vi "Feature_flower(SubVI).vi"(4 "黄色分量（油菜花）二值图":T1) -> (0 "SF 3":dbl, 1 "IFD 2":sgl, 2 "SFD 2":sgl, 3 "SH 2":dbl, 5 "SW 2":dbl, 7 "SE 2":dbl, 8 "SA":dbl)   [LabVIEW 2015]
uses:
  <vilib>/vision/Image Controls.llb/IMAQ Image.ctl
  <vilib>/vision/NI_Vision_Development_Module.lvlib
  2-top_features_oilseed/fractaldim.dll
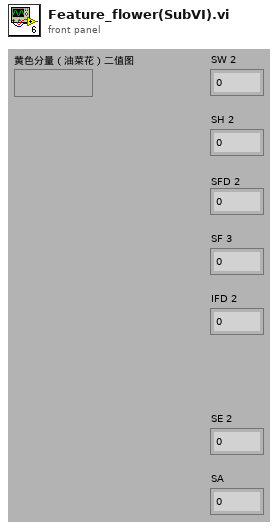
[diagram p1: front panel]
types:
  T1 = typedef "IMAQ Image.ctl" = refnum<image>
  T2 = typedef "Image Type" = u32
  T3 = typedef "Particle Parameters" = i32
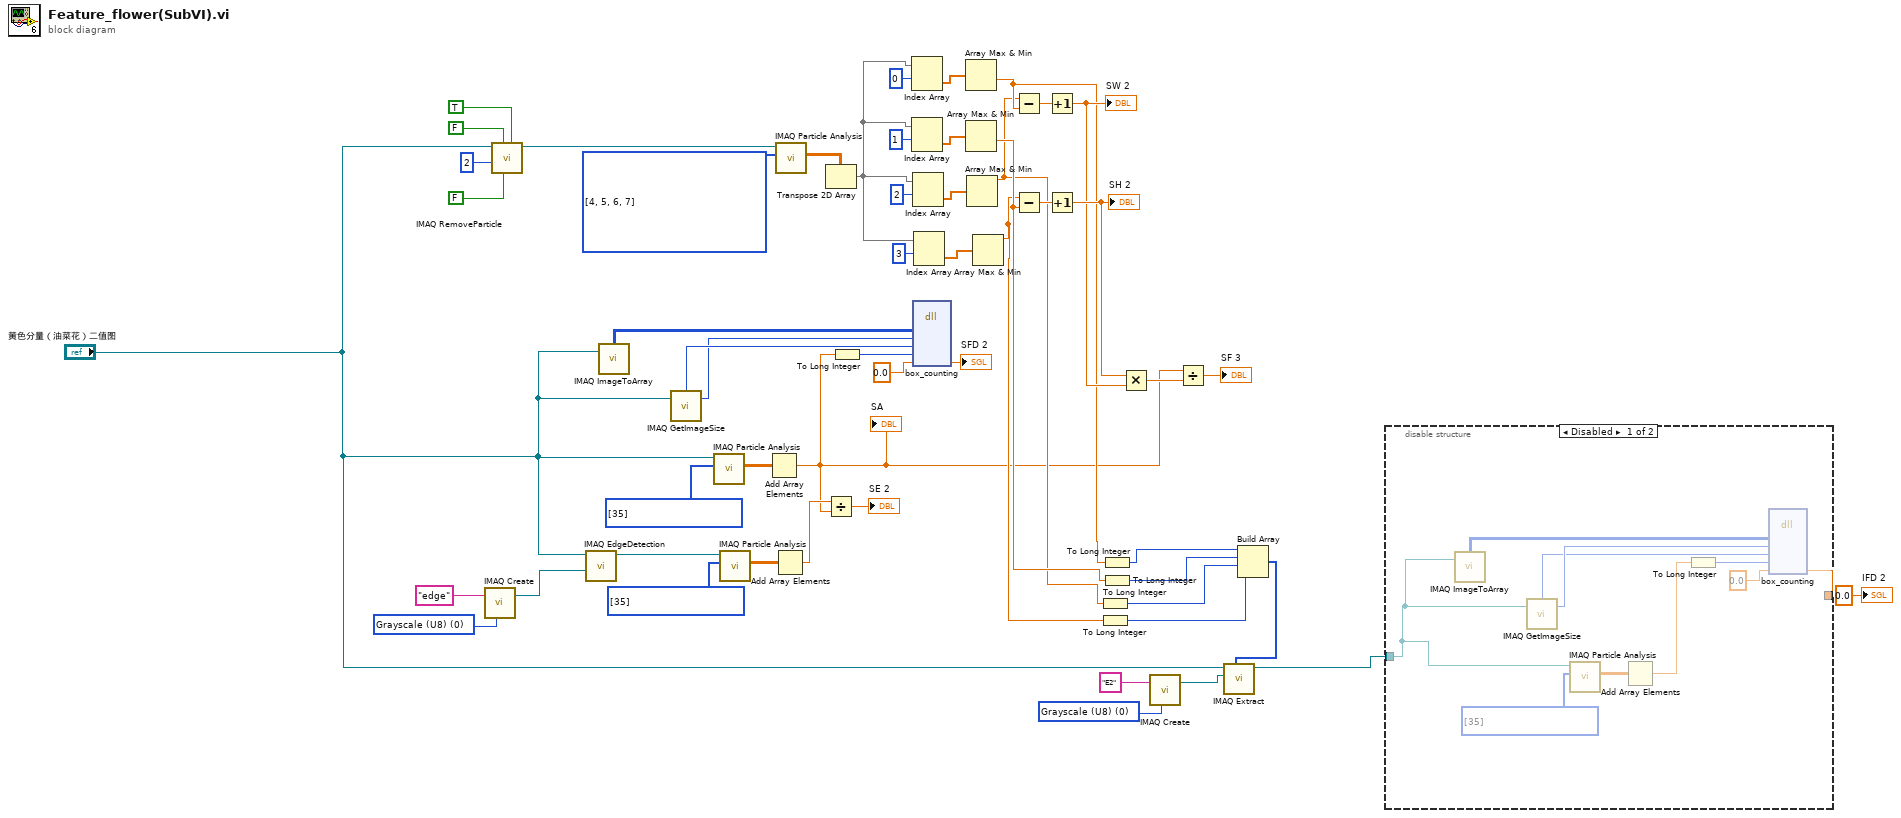
[diagram p0: block diagram]
diagram:
  w21 = T2 0 items=["Grayscale (U8)", "Grayscale (I16)", "Grayscale (SGL)", "Complex (CSG)", "RGB (U32)", "HSL (U32)", "RGB (U64)", "Grayscale (U16)"] ("Image Type")
  w38 = T3[] [4, 5, 6, 7] items=["Center of Mass X", "Center of Mass Y", "First Pixel X", "First Pixel Y", "Bounding Rect Left", "Bounding Rect Top", "Bounding Rect Right", "Bounding Rect Bottom", "Max Feret Diameter Start X", "Max Feret Diameter Start Y", "Max Feret Diameter End X", "Max Feret Diameter End Y", "Max Horiz. Segment Length Left", "Max Horiz. Segment Length Right", "Max Horiz. Segment Length Row", "-", "Bounding Rect Width", "Bounding Rect Height", "Bounding Rect Diagonal", "Perimeter", "Convex Hull Perimeter", "Holes' Perimeter", "Max Feret Diameter", "Equivalent Ellipse Major Axis", "Equivalent Ellipse Minor Axis", "Equivalent Ellipse Minor Axis (Feret)", "Equivalent Rect Long Side", "Equivalent Rect Short Side", "Equivalent Rect Diagonal", "Equivalent Rect Short Side (Feret)", "Average Horiz. Segment Length", "Average Vert. Segment Length", "Hydraulic Radius", "Waddel Disk Diameter", "-", "Area", "Holes' Area", "Particle & Holes' Area", "Convex Hull Area", "Image Area", "-", "Number of Holes", "Number of Horiz. Segments", "Number of Vert. Segments", "-", "Orientation", "Max Feret Diameter Orientation", "-", "% Area/Image Area", "% Area/(Particle & Holes' Area)", "Ratio of Equivalent Ellipse Axes", "Ratio of Equivalent Rect Sides", "-", "Elongation Factor", "Compactness Factor", "Heywood Circularity Factor", "Type Factor", "-", "Sum X", "Sum Y", "Sum XX", "Sum XY", "Sum YY", "Sum XXX", "Sum XXY", "Sum XYY", "Sum YYY", "-", "Moment of Inertia XX", "Moment of Inertia XY", "Moment of Inertia YY", "Moment of Inertia XXX", "Moment of Inertia XXY", "Moment of Inertia XYY", "Moment of Inertia YYY", "Norm. Moment of Inertia XX", "Norm. Moment of Inertia XY", "Norm. Moment of Inertia YY", "Norm. Moment of Inertia XXX", "Norm. Moment of Inertia XXY", "Norm. Moment of Inertia XYY", "Norm. Moment of Inertia YYY", "Hu Moment 1", "Hu Moment 2", "Hu Moment 3", "Hu Moment 4", "Hu Moment 5", "Hu Moment 6", "Hu Moment 7"] ("Pixel Measurements")
  w47 = T3[] [35] items=["Center of Mass X", "Center of Mass Y", "First Pixel X", "First Pixel Y", "Bounding Rect Left", "Bounding Rect Top", "Bounding Rect Right", "Bounding Rect Bottom", "Max Feret Diameter Start X", "Max Feret Diameter Start Y", "Max Feret Diameter End X", "Max Feret Diameter End Y", "Max Horiz. Segment Length Left", "Max Horiz. Segment Length Right", "Max Horiz. Segment Length Row", "-", "Bounding Rect Width", "Bounding Rect Height", "Bounding Rect Diagonal", "Perimeter", "Convex Hull Perimeter", "Holes' Perimeter", "Max Feret Diameter", "Equivalent Ellipse Major Axis", "Equivalent Ellipse Minor Axis", "Equivalent Ellipse Minor Axis (Feret)", "Equivalent Rect Long Side", "Equivalent Rect Short Side", "Equivalent Rect Diagonal", "Equivalent Rect Short Side (Feret)", "Average Horiz. Segment Length", "Average Vert. Segment Length", "Hydraulic Radius", "Waddel Disk Diameter", "-", "Area", "Holes' Area", "Particle & Holes' Area", "Convex Hull Area", "Image Area", "-", "Number of Holes", "Number of Horiz. Segments", "Number of Vert. Segments", "-", "Orientation", "Max Feret Diameter Orientation", "-", "% Area/Image Area", "% Area/(Particle & Holes' Area)", "Ratio of Equivalent Ellipse Axes", "Ratio of Equivalent Rect Sides", "-", "Elongation Factor", "Compactness Factor", "Heywood Circularity Factor", "Type Factor", "-", "Sum X", "Sum Y", "Sum XX", "Sum XY", "Sum YY", "Sum XXX", "Sum XXY", "Sum XYY", "Sum YYY", "-", "Moment of Inertia XX", "Moment of Inertia XY", "Moment of Inertia YY", "Moment of Inertia XXX", "Moment of Inertia XXY", "Moment of Inertia XYY", "Moment of Inertia YYY", "Norm. Moment of Inertia XX", "Norm. Moment of Inertia XY", "Norm. Moment of Inertia YY", "Norm. Moment of Inertia XXX", "Norm. Moment of Inertia XXY", "Norm. Moment of Inertia XYY", "Norm. Moment of Inertia YYY", "Hu Moment 1", "Hu Moment 2", "Hu Moment 3", "Hu Moment 4", "Hu Moment 5", "Hu Moment 6", "Hu Moment 7"] ("Pixel Measurements")
  w50 = T2 0 items=["Grayscale (U8)", "Grayscale (I16)", "Grayscale (SGL)", "Complex (CSG)", "RGB (U32)", "HSL (U32)", "RGB (U64)", "Grayscale (U16)"] ("Image Type")
  w53 = T3[] [35] items=["Center of Mass X", "Center of Mass Y", "First Pixel X", "First Pixel Y", "Bounding Rect Left", "Bounding Rect Top", "Bounding Rect Right", "Bounding Rect Bottom", "Max Feret Diameter Start X", "Max Feret Diameter Start Y", "Max Feret Diameter End X", "Max Feret Diameter End Y", "Max Horiz. Segment Length Left", "Max Horiz. Segment Length Right", "Max Horiz. Segment Length Row", "-", "Bounding Rect Width", "Bounding Rect Height", "Bounding Rect Diagonal", "Perimeter", "Convex Hull Perimeter", "Holes' Perimeter", "Max Feret Diameter", "Equivalent Ellipse Major Axis", "Equivalent Ellipse Minor Axis", "Equivalent Ellipse Minor Axis (Feret)", "Equivalent Rect Long Side", "Equivalent Rect Short Side", "Equivalent Rect Diagonal", "Equivalent Rect Short Side (Feret)", "Average Horiz. Segment Length", "Average Vert. Segment Length", "Hydraulic Radius", "Waddel Disk Diameter", "-", "Area", "Holes' Area", "Particle & Holes' Area", "Convex Hull Area", "Image Area", "-", "Number of Holes", "Number of Horiz. Segments", "Number of Vert. Segments", "-", "Orientation", "Max Feret Diameter Orientation", "-", "% Area/Image Area", "% Area/(Particle & Holes' Area)", "Ratio of Equivalent Ellipse Axes", "Ratio of Equivalent Rect Sides", "-", "Elongation Factor", "Compactness Factor", "Heywood Circularity Factor", "Type Factor", "-", "Sum X", "Sum Y", "Sum XX", "Sum XY", "Sum YY", "Sum XXX", "Sum XXY", "Sum XYY", "Sum YYY", "-", "Moment of Inertia XX", "Moment of Inertia XY", "Moment of Inertia YY", "Moment of Inertia XXX", "Moment of Inertia XXY", "Moment of Inertia XYY", "Moment of Inertia YYY", "Norm. Moment of Inertia XX", "Norm. Moment of Inertia XY", "Norm. Moment of Inertia YY", "Norm. Moment of Inertia XXX", "Norm. Moment of Inertia XXY", "Norm. Moment of Inertia XYY", "Norm. Moment of Inertia YYY", "Hu Moment 1", "Hu Moment 2", "Hu Moment 3", "Hu Moment 4", "Hu Moment 5", "Hu Moment 6", "Hu Moment 7"] ("Pixel Measurements")
  n1 = call "IMAQ Create"("Image Name"="edge", "Image Type"=w50) -> ("New Image"=w49:T1)  [unwired: 2 in, 2 out]
  n2 = call "IMAQ RemoveParticle"("Connectivity 4/8 (8)"=TRUE, "Low Pass/High Pass (Low)"=FALSE, "Square/Hexa (Square)"=FALSE, "Number of Erosion"=2, "Image Src"="黄色分量（油菜花）二值图") -> ("Image Dst Out"=w3:T1)  [unwired: 2 in, 4 out]
  n3 = call "IMAQ EdgeDetection"("Image Dst"=w49, "Image Src"="黄色分量（油菜花）二值图") -> ("Image Dst Out"=w52:T1)  [unwired: 4 in, 5 out]
  n4 = call "IMAQ ImageToArray"("Image"="黄色分量（油菜花）二值图") -> ("Image Pixels (U8)"=w43:u8[][])  [unwired: 2 in, 5 out]
  n5 = call "IMAQ GetImageSize"("Image"="黄色分量（油菜花）二值图") -> ("Y Resolution"=w39:i32, "X Resolution"=w40:i32)  [unwired: 1 in, 3 out]
  n6 = call "IMAQ Particle Analysis"("Pixel Measurements"=w47, "Image"="黄色分量（油菜花）二值图") -> ("Particle Measurements (Pixels)"=w48:dbl[][])  [unwired: 3 in, 6 out]
  n7 = call "IMAQ Particle Analysis"("Pixel Measurements"=w53, "Image"=w52) -> ("Particle Measurements (Pixels)"=w54:dbl[][])  [unwired: 3 in, 6 out]
  n8 = Add Array Elements(numeric array=w48) -> (sum=w8:dbl)
  "SA" <- w8
  n9 = Add Array Elements(numeric array=w54) -> (sum=w46:dbl)
  n10 = call "IMAQ Particle Analysis"("Pixel Measurements"=w38, "Image"=w3) -> ("Particle Measurements (Pixels)"=w37:dbl[][])  [unwired: 3 in, 6 out]
  n11 = Transpose 2D Array(2D array=w37) -> (transposed array=w28:dbl[][])
  n12 = Divide(x=w46, y=w8) -> (x/y=→"SE 2":dbl)
  n13 = To Long Integer(number=w8) -> (32bit integer=w42:i32)
  n14 = Index Array(array=w28, index (row)=0) -> (element=w30:dbl[])  [unwired: 1 in]
  n15 = Index Array(array=w28, index (row)=1) -> (element=w31:dbl[])  [unwired: 1 in]
  n16 = Index Array(array=w28, index (row)=2) -> (element=w35:dbl[])  [unwired: 1 in]
  n17 = dll-call lib="H:/2-top_features_oilseed/fractaldim.dll" fn="box_counting"("bw"=w43, "row"=w39, "col"=w40, "area"=w42, "FD"=sgl 0.0) -> ("FD"=→"SFD 2":sgl)  [unwired: 7 in, 3 out]
  n18 = Index Array(array=w28, index (row)=3) -> (element=w34:dbl[])  [unwired: 1 in]
  n19 = Array Max & Min(array=w30) -> (min value=w18:dbl)  [unwired: 3 out]
  n20 = Array Max & Min(array=w31) -> (min value=w16:dbl)  [unwired: 3 out]
  n21 = Array Max & Min(array=w35) -> (max value=w14:dbl)  [unwired: 3 out]
  n22 = Array Max & Min(array=w34) -> (max value=w12:dbl)  [unwired: 3 out]
  n23 = Subtract(x=w14, y=w18) -> (x-y=w27:dbl)
  n24 = Subtract(x=w12, y=w16) -> (x-y=w26:dbl)
  n25 = Increment(x=w27) -> (x+1=w23:dbl)
  "SW 2" <- w23
  n26 = Increment(x=w26) -> (x+1=w24:dbl)
  "SH 2" <- w24
  n27 = To Long Integer(number=w14) -> (32bit integer=w13:i32)
  n28 = To Long Integer(number=w12) -> (32bit integer=w11:i32)
  n29 = To Long Integer(number=w18) -> (32bit integer=w17:i32)
  n30 = To Long Integer(number=w16) -> (32bit integer=w15:i32)
  n31 = Multiply(x=w24, y=w23) -> (x*y=w25:dbl)
  n32 = call "IMAQ Create"("Image Name"="E2", "Image Type"=w21) -> ("New Image"=w19:T1)  [unwired: 2 in, 2 out]
  n33 = Divide(x=w8, y=w25) -> (x/y=→"SF 3":dbl)
  n34 = Build Array(w17, w15, w13, w11) -> (w10:i32[])
  n35 = call "IMAQ Extract"("Optional Rectangle"=w10, "Image Dst"=w19, "Image Src"="黄色分量（油菜花）二值图") -> ("Image Dst Out"=w9:T1)  [unwired: 3 in, 5 out]
  n36 = disable-structure shown="Disabled" {
    disable-tunnel: [w61 _] -> _
    disable-tunnel: w9 -> [w55 _]
    frame Disabled {
      w57 = T3[] [35] items=["Center of Mass X", "Center of Mass Y", "First Pixel X", "First Pixel Y", "Bounding Rect Left", "Bounding Rect Top", "Bounding Rect Right", "Bounding Rect Bottom", "Max Feret Diameter Start X", "Max Feret Diameter Start Y", "Max Feret Diameter End X", "Max Feret Diameter End Y", "Max Horiz. Segment Length Left", "Max Horiz. Segment Length Right", "Max Horiz. Segment Length Row", "-", "Bounding Rect Width", "Bounding Rect Height", "Bounding Rect Diagonal", "Perimeter", "Convex Hull Perimeter", "Holes' Perimeter", "Max Feret Diameter", "Equivalent Ellipse Major Axis", "Equivalent Ellipse Minor Axis", "Equivalent Ellipse Minor Axis (Feret)", "Equivalent Rect Long Side", "Equivalent Rect Short Side", "Equivalent Rect Diagonal", "Equivalent Rect Short Side (Feret)", "Average Horiz. Segment Length", "Average Vert. Segment Length", "Hydraulic Radius", "Waddel Disk Diameter", "-", "Area", "Holes' Area", "Particle & Holes' Area", "Convex Hull Area", "Image Area", "-", "Number of Holes", "Number of Horiz. Segments", "Number of Vert. Segments", "-", "Orientation", "Max Feret Diameter Orientation", "-", "% Area/Image Area", "% Area/(Particle & Holes' Area)", "Ratio of Equivalent Ellipse Axes", "Ratio of Equivalent Rect Sides", "-", "Elongation Factor", "Compactness Factor", "Heywood Circularity Factor", "Type Factor", "-", "Sum X", "Sum Y", "Sum XX", "Sum XY", "Sum YY", "Sum XXX", "Sum XXY", "Sum XYY", "Sum YYY", "-", "Moment of Inertia XX", "Moment of Inertia XY", "Moment of Inertia YY", "Moment of Inertia XXX", "Moment of Inertia XXY", "Moment of Inertia XYY", "Moment of Inertia YYY", "Norm. Moment of Inertia XX", "Norm. Moment of Inertia XY", "Norm. Moment of Inertia YY", "Norm. Moment of Inertia XXX", "Norm. Moment of Inertia XXY", "Norm. Moment of Inertia XYY", "Norm. Moment of Inertia YYY", "Hu Moment 1", "Hu Moment 2", "Hu Moment 3", "Hu Moment 4", "Hu Moment 5", "Hu Moment 6", "Hu Moment 7"] ("Pixel Measurements")
      n37 = call "IMAQ ImageToArray"("Image"=w55) -> ("Image Pixels (U8)"=w59:u8[][])  [unwired: 2 in, 5 out]
      n38 = call "IMAQ GetImageSize"("Image"=w55) -> ("Y Resolution"=w63:i32, "X Resolution"=w62:i32)  [unwired: 1 in, 3 out]
      n39 = call "IMAQ Particle Analysis"("Pixel Measurements"=w57, "Image"=w55) -> ("Particle Measurements (Pixels)"=w56:dbl[][])  [unwired: 3 in, 6 out]
      n40 = Add Array Elements(numeric array=w56) -> (sum=w64:dbl)
      n41 = To Long Integer(number=w64) -> (32bit integer=w60:i32)
      n42 = dll-call lib="H:/2-top_features_oilseed/fractaldim.dll" fn="box_counting"("bw"=w59, "row"=w63, "col"=w62, "area"=w60, "FD"=sgl 0.0) -> ("FD"=w61:sgl)  [unwired: 7 in, 3 out]
    }
    frame Enabled {
    }
  }
  "IFD 2" <- sgl 0.0 ("IFD 2")
